vi "Get Default Timeout.vi"() -> (3 "default timeout (ms)":i32)   [LabVIEW 2020, in "NI_WFCN.lvlib"]
doc: "Returns a suggested timeout value for Wait for Configured Network."
uses:
  <vilib>/net/WFCN/NI_WFCN.lvlib
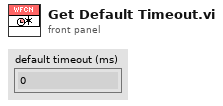
[diagram p1: front panel]
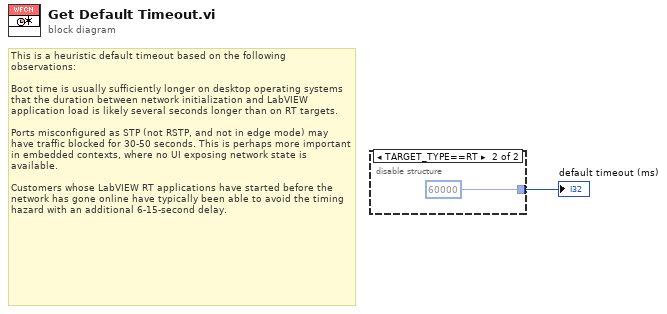
[diagram p0: block diagram]
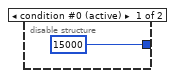
[diagram p2: hidden frame]
diagram:
  # "This is a heuristic default timeout based on the following observations:\n\nBoot time is usually sufficiently longer on desktop operating systems that the duration between network initialization and LabVIEW application load is likely several seconds longer than on RT targets.\n\nPorts misconfigured as STP (not RSTP, and not in edge mode) may have traffic blocked for 30-50 seconds. This is perhaps more important in embedded contexts, where no UI exposing network state is available.\n\nCustomers whose LabVIEW RT applications have started before the network has gone online have typically been able to avoid the timing hazard with an additional 6-15-second delay."
  n1 = disable-structure shown="TARGET_TYPE==RT" {
    disable-tunnel: [15000 60000] -> w1
    frame condition #0 (active) {
    }
    frame condition #1 {
    }
  }
  "default timeout (ms)" <- w1
